vi "Setup.vi"(8 "error in (no error)":errorcluster, 11 "XML Report Test In":refnum<class "Text Report Test.lvclass">) -> (0 "error out":errorcluster, 3 "XML Report Test Out":refnum<class "Text Report Test.lvclass">)   [LabVIEW 2020, in "Text Report Test.lvclass"]
doc: "Setup method called by the testing framework before each test method is called."
uses:
  Text Report Test.lvclass
  Text Report Test.lvclass/Text Report Test.ctl
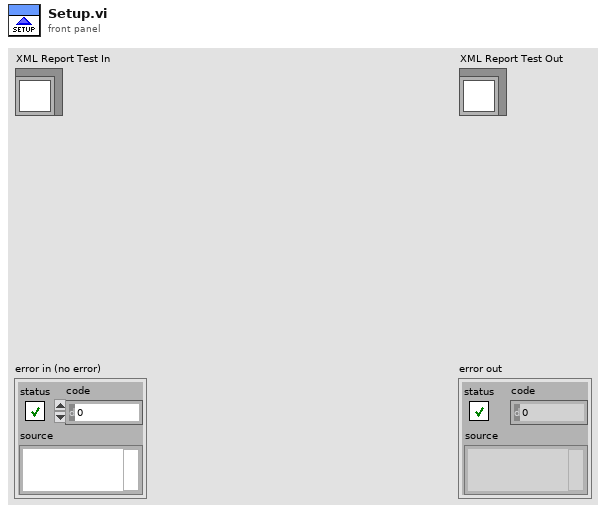
[diagram p1: front panel]
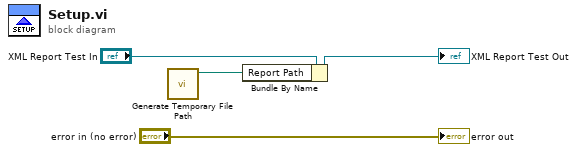
[diagram p0: block diagram]
diagram:
  n1 = call <vilib>:"Generate Temporary File Path.vi"() -> ("Unique Temporary File Path"=w1:path)  [unwired: 10 in, 1 out]
  n2 = Bundle By Name(cluster="XML Report Test In", "Report Path"=w1) -> (→"XML Report Test Out":refnum<class "Text Report Test.lvclass">)
  "error out" <- "error in (no error)"
